vi "Get string array size without blanks.vi"(2 "String array":string[](array[string])) -> (14 "Corrected array size":i32=1 min=0 max=20 step=1)   [LabVIEW 2020]
doc: "This VI returns the size of a string array without counting white space strings."
panel:
  # "Returns the size of a string array\nwithout counting white space strings."
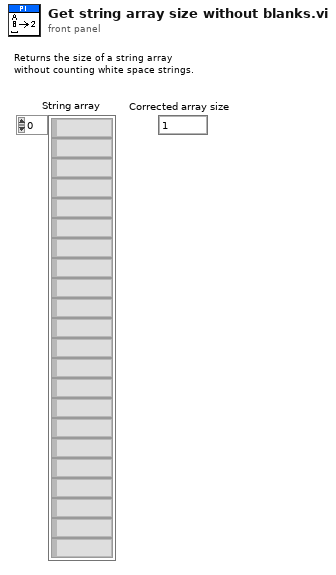
[diagram p1: front panel]
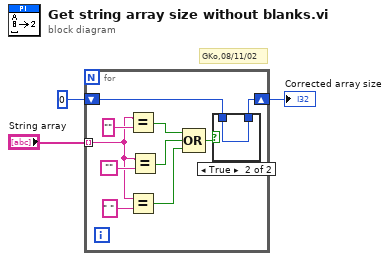
[diagram p0: block diagram]
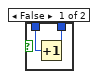
[diagram p2: hidden frame]
diagram:
  # "GKo,08/11/02"
  n1 = for {
    tunnel: "String array" -> [w10] mode=indexing
    shift-right: [w4] -> w1
    shift-left: 0 -> [w5]
    n2 = Equal?(x=w10, y="") -> (x = y?=w9:bool)
    n3 = Equal?(x=w10, y=" ") -> (x = y?=w7:bool)
    n4 = Equal?(x=w10, y="") -> (x = y?=w8:bool)
    n5 = Compound Arithmetic op=OR(w9, w8, w7) -> (w6:bool)
    n6 = case shown="True" w6 {
      tunnel: w5 -> [w15 w16]
      tunnel: [w14 w16] -> w4
      frame False {
        n7 = Increment(x=w15) -> (x+1=w14:i32)
      }
      frame True {
      }
    }
  }
  "Corrected array size" <- w1
